vi "Get Laser Drive.vi"(8 "error in (no error)":errorcluster, 9 "Path":path, 10 "Section":string, 11 "Sim Laser Factory in":refnum<class "Sim Laser Factory.lvclass">) -> (0 "error out":errorcluster, 2 "Laser Driver.lvclass":refnum<class "Laser Driver.lvclass">)   [LabVIEW 2022 SP3, in "Sim Laser Factory.lvclass"]
uses:
  Sim Laser Factory.lvclass
  Sim Laser Factory.lvclass/Sim Laser Factory.ctl
  Sim Laser Driver/Sim Laser Driver.lvclass
  C:/XY Stage/XY Stage/Framework/Base/Base.lvclass
  C:/XY Stage/Laser/Sim Laser Driver/Sim Laser Driver.lvclass
  C:/XY Stage/Laser/Laser Driver/Laser Driver.lvclass
  Laser Driver/Laser Driver.lvclass
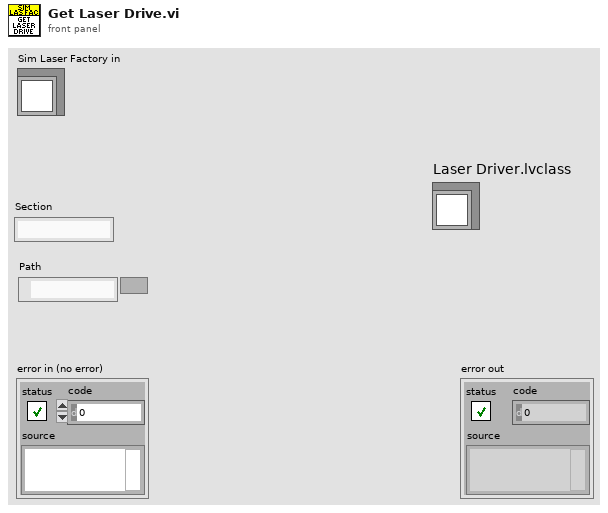
[diagram p1: front panel]
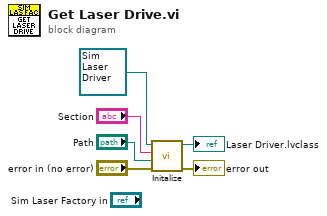
[diagram p0: block diagram]
diagram:
  n1 = call "Initalize.vi"("error in (no error)"="error in (no error)", "Path"="Path", "Section"="Section", "Sim Laser Driver in"=refnum<class "Sim Laser Driver.lvclass"> refnum ("Sim Laser Driver.lvclass")) -> ("error out"=→"error out":errorcluster, "Sim Laser Driver out"=→"Laser Driver.lvclass":refnum<class "Sim Laser Driver.lvclass">)  [unwired: 6 in]
